vi "setFilePath(Dialog if necessary).vi"(8 "error in (no error)":errorcluster, 10 "FilePath":path, 11 "Document in":refnum<class "Document.lvclass">) -> (0 "error out":errorcluster, 3 "Document out":refnum<class "Document.lvclass">)   [LabVIEW 2020, in "LabVIEW NPOI.lvlib" / "Document.lvclass"]
doc: "Sets the <b>File Path</b> from the <b>Document</b>.\n\nNotes:\n - If <b>File Path</b> is empty (default) or is <Not A Path> or is a directory, the VI displays a dialog box from which the user can select a file. Error 43 occurs if you cancel the dialog box. \n - If the <b>File Path</b> already contains a docuement with the same name then that file is overwritten without warning."
uses:
  Document.lvclass
  Document.lvclass/Document.ctl
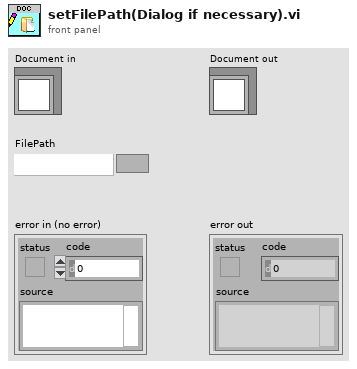
[diagram p1: front panel]
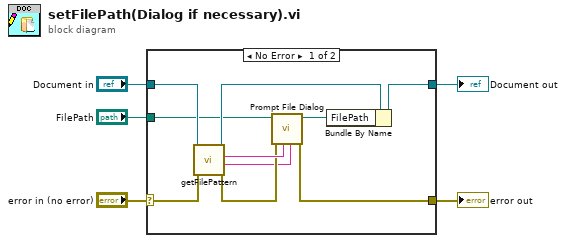
[diagram p0: block diagram]
diagram:
  n1 = case shown="No Error" "error in (no error)" {
    selector: "error in (no error)" -> [w9 w16]
    tunnel: [w13 w16] -> w4
    tunnel: [w15 w17] -> w2
    tunnel: "Document in" -> [w12 w17]
    tunnel: "FilePath" -> [w6 _]
    frame No Error {
      n2 = call-dynamic "getFilePattern.vi"("error in (no error)"=w9, "Document in"=w12) -> ("error out"=w8:errorcluster, "pattern"=w7:string, "pattern label"=w10:string, "Document out"=w11:refnum<class "Document.lvclass">)  [unwired: 6 in]
      n3 = call "Prompt File Dialog.vi"("pattern (all files)"=w7, "pattern label"=w10, "error in"=w8, "File Path"=w6) -> ("error out"=w13:errorcluster, "selected path"=w14:path)  [unwired: 6 in]
      n4 = Bundle By Name(cluster=w11, "FilePath"=w14) -> (w15:refnum<class "Document.lvclass">)
    }
    frame Error {
    }
  }
  "error out" <- w4
  "Document out" <- w2
